vi "rdb_json_decode_string.vi"(8 "error in (no error)":errorcluster, 9 "offset (0)":i32, 11 "json":string) -> (0 "error out":errorcluster, 1 "offset past match":i32, 2 "value":variant, 3 "type":T1)   [LabVIEW 2017]
uses:
  rdb_json_type.ctl
  <vilib>/Utility/error.llb/Error Cluster From Error Code.vi
  <vilib>/regexp/Match Regular Expression.xnode
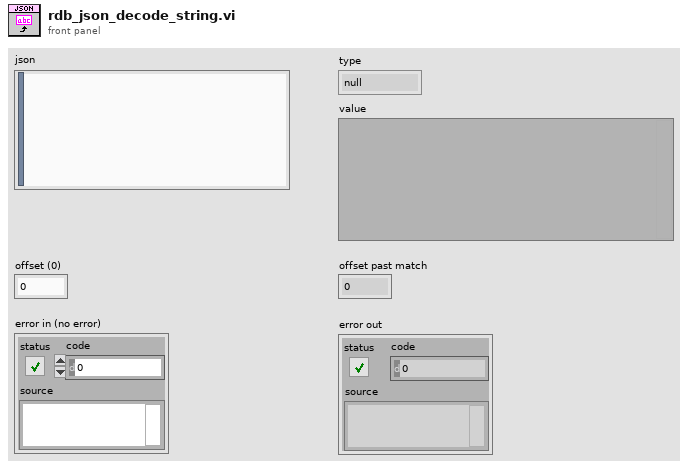
[diagram p1: front panel]
types:
  T1 = typedef "rdb_json_type.ctl" = enum8{"null", "bool", "int", "uint", "float", "string", "array", "object", "invalid"}
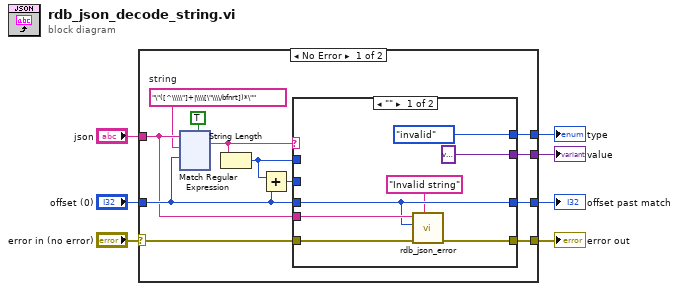
[diagram p0: block diagram]
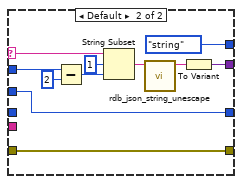
[diagram p2: hidden frame]
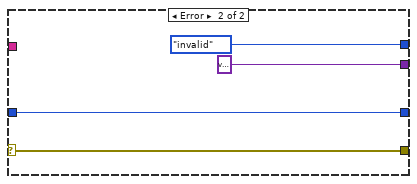
[diagram p3: hidden frame]
diagram:
  n1 = case shown="No Error" "error in (no error)" {
    selector: "error in (no error)" -> [w18 w155]
    tunnel: "json" -> [w11 _]
    tunnel: [w19 w155] -> w6
    tunnel: "offset (0)" -> [w13 w154]
    tunnel: [w17 w154] -> w3
    tunnel: [w16 rdb_json_type."invalid" ("type")] -> w2
    tunnel: [w15 variant ("Variant")] -> w1
    frame No Error {
      w9 = "\"([^\\\\\"]+|\\\\[\"\\\\/bfnrt])*\""  # string
      n2 = xnode "Match Regular Expression"("input string"=w11, "regular expression"=w9, "offset (0)"=w13, "multiline? (F)"=TRUE) -> ("whole match"=w12:string)  [unwired: 2 in, 4 out]
      n3 = String Length(string=w12) -> (length=w10:i32)
      n4 = Add(x=w10, y=w13) -> (x+y=w14:i32)
      n5 = case shown="\"\"" w12 {
        selector: w12 -> [_ w143]
        tunnel: w13 -> [w136 _]
        tunnel: [w135 w149] -> w19
        tunnel: w18 -> [w138 w149]
        tunnel: [w136 w148] -> w17
        tunnel: [rdb_json_type."invalid" ("type") rdb_json_type."string" ("type")] -> w16
        tunnel: [variant ("Variant") w150] -> w15
        tunnel: w14 -> [_ w148]
        tunnel: w11 -> [w137 _]
        tunnel: w10 -> [_ w142]
        frame "" {
          n6 = call "rdb_json_error.vi"("message"="Invalid string" ("error message (\"\")"), "error in (no error)"=w138, "offset (0)"=w136, "json"=w137) -> ("error out"=w135:errorcluster)  [unwired: 7 in]
        }
        frame Default {
          n7 = Subtract(x=w142, y=2) -> (x-y=w144:i32)
          n8 = String Subset(string=w143, offset (0)=1, length (rest)=w144) -> (substring=w147:string)
          n9 = call "rdb_json_string_unescape.vi"("escaped string"=w147) -> ("string out"=w141:string)  [unwired: 9 in, 1 out]
          n10 = To Variant(anything=w141) -> (Variant=w150:variant)
        }
      }
    }
    frame Error {
    }
  }
  "error out" <- w6
  "offset past match" <- w3
  "type" <- w2
  "value" <- w1
